vi "SMART__Yt13_SimpleGenericTest.vi"() -> ()   [LabVIEW 2017]
uses:
  Step`s VIs/YYLLIdea/yylltestresult/yylltestresult basis.ctl
  <vilib>/Utility/miscctls.llb/LVPointTypeDef.ctl
  <vilib>/Instr/_visa.llb/VISA Configure Serial Port (Instr).vi
panel:
  in  "Hex?(StringLimit-A)":bool caption="Hex?"
  in  "Hex?(接收解析后)":bool caption="Hex?"
  in  "Hex?(最终发送)":bool caption="Hex?"
  in  "真发送并获取接收的":bool
  in  "解析后到变量(自定义建议#开头)":string(combo)="不到变量"
  in  "明码LOG":bool
  in  "unit":string
  out "WaitTime":u32 format="%dms"
  in  "打开串口":bool
  in  "baud rate":string(combo)="9600"
  in  "应答≥长度检测":i32
  in  "应答检测":string
  in  "Hex?(假设接收)":bool caption="Hex?"
  out "结果预览":bool
  in  "LowLimit-C":dbl
  in  "UpperLimit-B":dbl
  in  "StringLimit-A":string
  in  "合格依据":T1 caption="Enum 3"
  in  "假设、收到的\n字符串":string
  out "解析后":string
  in  "Smart解析预处理btn":bool
  out "最终发送":string
  in  "发送字符串":string
  in  "Smart发送预处理btn":bool
  in  "Smart解析预处理":string[][](array[string])
  in  "Smart发送预处理":string[][](array[string])
  in  "VISA resource":refnum<visa-resource-name>
  in  "接收前延迟ms":u32
  in  "接收延迟前&发送前清缓存":bool=TRUE
  in  "Hex?(发送)":bool caption="Hex?"
  # "yyllSerial.SimpleTest"
  # "需提前运行好串口配置步骤！或这里临时打开"
  # "注意自收发参与统计"
  # "解析后：\nX值 ->"
  # "#yylltips:要判断MAC可以通过正则“\\w{12}”"
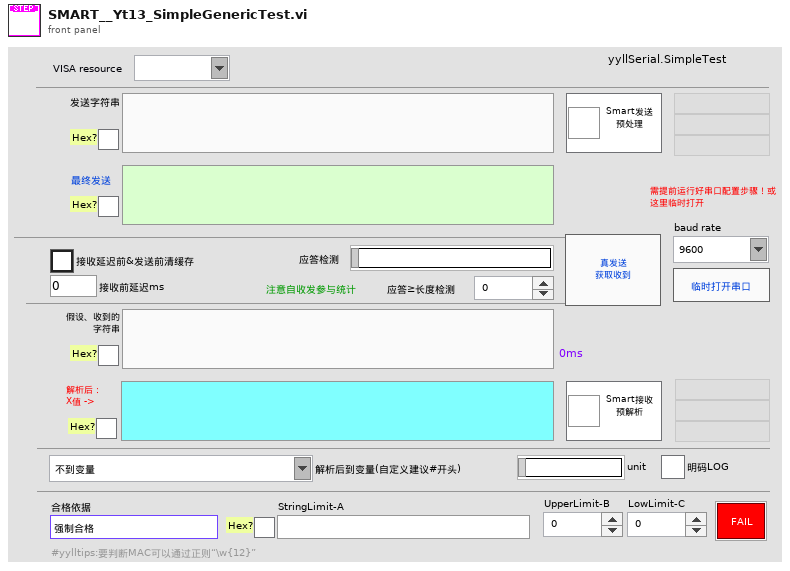
[diagram p1: front panel]
types:
  T1 = typedef "yylltestresult basis.ctl" = enum16{"强制合格", "强制不合格", "随机合格", "X=A", "X=\"真\"", "X=\"假\"", "X≠A", "X包含A", "X不包含A", "A包含X", "A包含非空X", "A不包含X", "X等于A正则匹配内容", "X包含A正则匹配内容", "X不包含A正则匹配内容", "X=B", "X≠B", "X＞B", "X≥B", "X＜B", "X≤B", "B≥X≥C", "B≥X＞C", "B＞X≥C", "B＞X＞C", "X≥B | C≥X", "X＞B | C≥X", "X≥B | C＞X", "X＞B | C＞X"}
  T2 = typedef "LVPointTypeDef.ctl" = cluster{"Horizontal":i16, "Vertical":i16}
  T3 = enum16{"open", "replace", "create", "open or create", "replace or create", "replace or create with confirmation"}
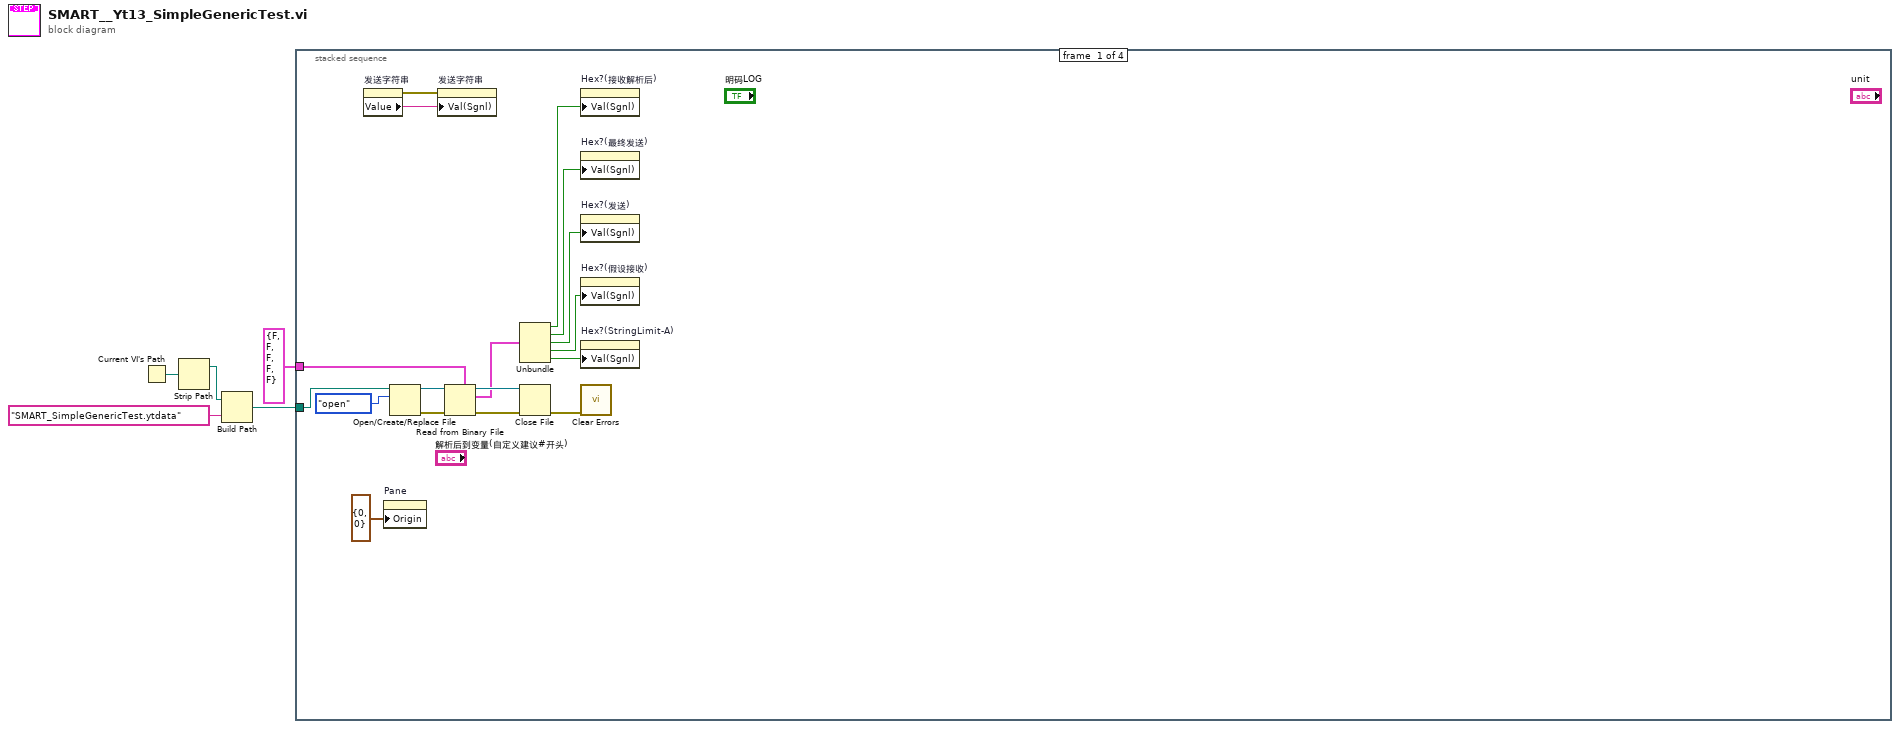
[diagram p0: block diagram]
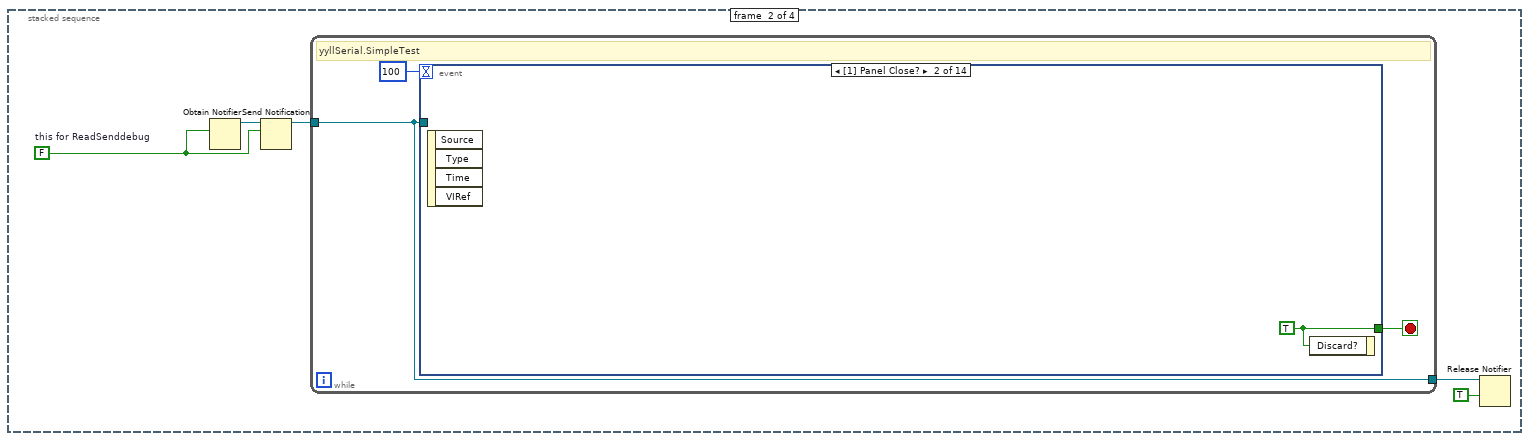
[diagram p2: hidden frame]
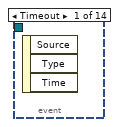
[diagram p3: hidden frame]
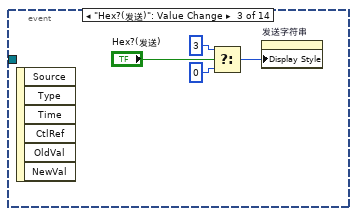
[diagram p4: hidden frame]
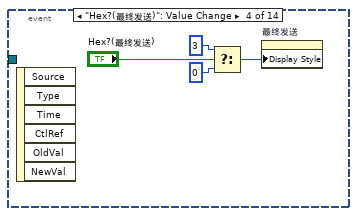
[diagram p5: hidden frame]
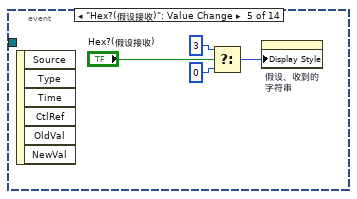
[diagram p6: hidden frame]
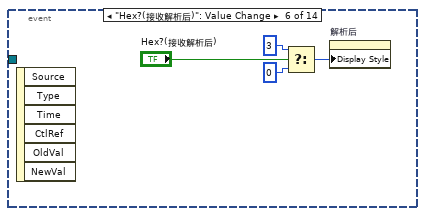
[diagram p7: hidden frame]
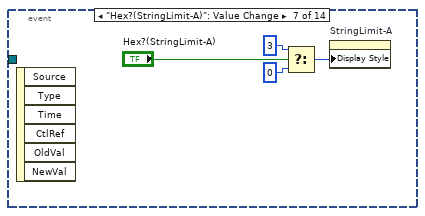
[diagram p8: hidden frame]
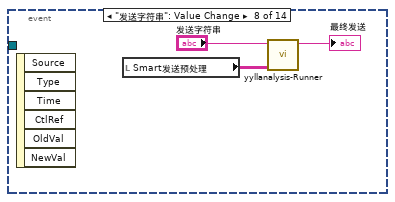
[diagram p9: hidden frame]
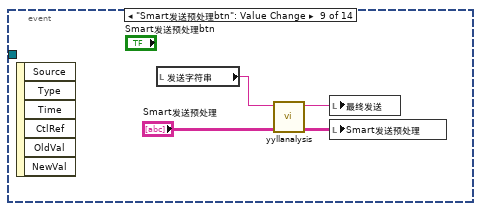
[diagram p10: hidden frame]
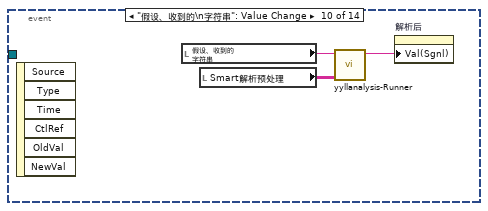
[diagram p11: hidden frame]
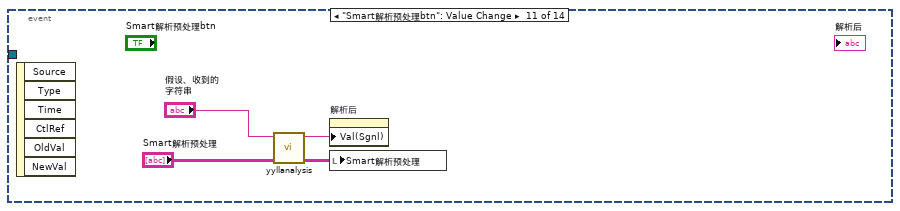
[diagram p12: hidden frame]
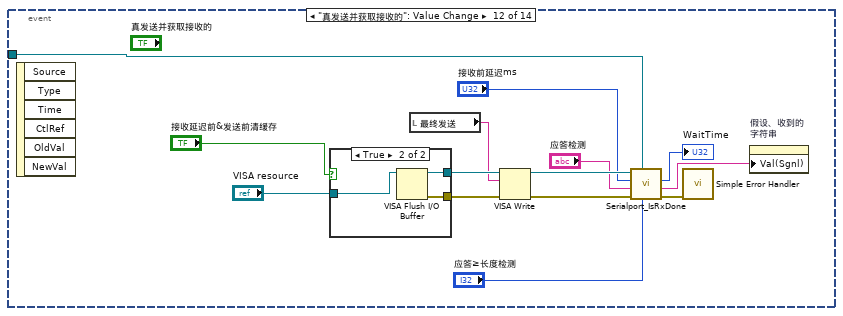
[diagram p13: hidden frame]
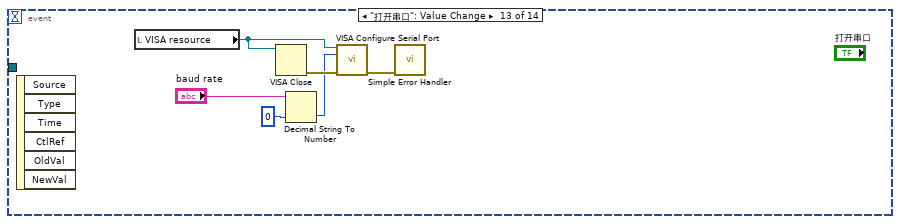
[diagram p15: hidden frame]
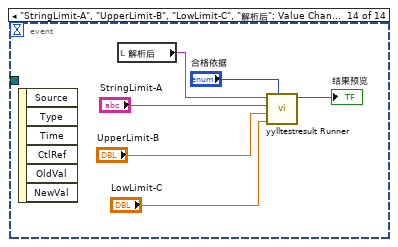
[diagram p16: hidden frame]
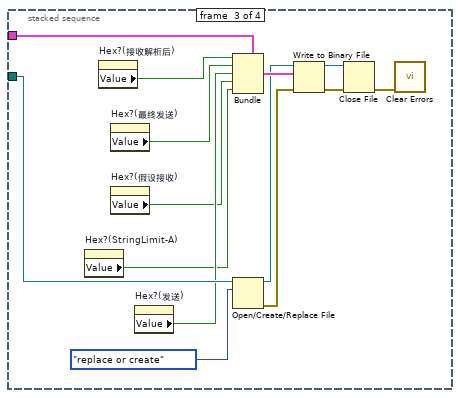
[diagram p17: hidden frame]
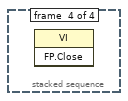
[diagram p18: hidden frame]
diagram:
  n1 = Current VI's Path() -> (path=w3:path)
  n2 = Strip Path(path=w3) -> (stripped path=w4:path)  [unwired: 1 out]
  n3 = Build Path(base path=w4, name or relative path="SMART_SimpleGenericTest.ytdata") -> (appended path=w2:path)
  n4 = stacked-sequence {
    tunnel: cluster{bool, bool, bool, bool, bool} {FALSE, FALSE, FALSE, FALSE, FALSE} -> [w9 _ w109 _]
    tunnel: w2 -> [w8 _ w108 _]
    frame #0 {
      n5 = property on="发送字符串" class="Str"() -> (error out=w22:errorcluster, "Value"=w21:string)  [unwired: 2 in, 1 out]
      n6 = property on="Pane" class="Pane"("Origin"=T2 {"Horizontal"=0, "Vertical"=0}) -> ()  [unwired: 2 in, 2 out]
      n7 = Open/Create/Replace File(file path (use dialog)=w8, operation (0:open)=T3."open") -> (refnum out=w12:refnum<file>, error out=w10:errorcluster)  [unwired: 4 in, 1 out]
      n8 = property on="发送字符串" class="Str"(error in=w22, "Val(Sgnl)"=w21) -> ()  [unwired: 1 in, 2 out]
      n9 = Read from Binary File(5:w9, 8:w10, 11:w12) -> (0:w13:errorcluster, 2:w14:cluster{bool, bool, bool, bool, bool}, 3:w20:refnum<file>)  [unwired: 3 in, 1 out]
      n10 = Unbundle(w14) -> (w19:bool, w18:bool, w17:bool, w16:bool, w15:bool)
      n11 = Close File(refnum=w20, error in=w13) -> (error out=w7:errorcluster)  [unwired: 1 out]
      n12 = property on="Hex?(接收解析后)" class="Bool (strict)"("Val(Sgnl)"=w19) -> ()  [unwired: 2 in, 2 out]
      n13 = property on="Hex?(最终发送)" class="Bool (strict)"("Val(Sgnl)"=w18) -> ()  [unwired: 2 in, 2 out]
      n14 = property on="Hex?(发送)" class="Bool (strict)"("Val(Sgnl)"=w17) -> ()  [unwired: 2 in, 2 out]
      n15 = property on="Hex?(假设接收)" class="Bool (strict)"("Val(Sgnl)"=w16) -> ()  [unwired: 2 in, 2 out]
      n16 = property on="Hex?(StringLimit-A)" class="Bool (strict)"("Val(Sgnl)"=w15) -> ()  [unwired: 2 in, 2 out]
      n17 = call <vilib>:"Clear Errors.vi"("error in (no error)"=w7) -> ()  [unwired: 5 in, 2 out]
    }
    frame #1 {
      w23 = FALSE  # this for ReadSenddebug
      n18 = Obtain Notifier(notification data type=w23) -> (notifier out=w25:refnum<notifier>)  [unwired: 3 in, 2 out]
      n19 = Send Notification(notification=w23, notifier=w25) -> (notifier out=w26:refnum<notifier>)  [unwired: 1 in, 1 out]
      n20 = while {
        tunnel: w26 -> [w28]
        tunnel: [w28] -> w27
        stop <- w29 stop-if-true
        # "yyllSerial.SimpleTest"
        n21 = event shown="[1] Panel Close?" {
          selector: _ -> [_ _ _ _ _ _ _ _ _ _ _ _ _ _]
          dyn-events: _ -> [_ _ _ _ _ _ _ _ _ _ _ _ _ _]
          timeout: 100 -> [_ _ _ _ _ _ _ _ _ _ _ _ _ _]
          tunnel: [_ w31 _ _ _ _ _ _ _ _ _ _ _ _] -> w29
          tunnel: w28 -> [_ _ _ _ _ _ _ _ _ _ _ w67 _ _]
          event Timeout {
            n22 = event-data() -> ()  [unwired: 1 in, 3 out]
          }
          event Panel Close? {
            w31 = TRUE
            n23 = event-data() -> ()  [unwired: 1 in, 4 out]
            n24 = event-data("Discard?"=w31) -> ()  [unwired: 1 in, 1 out]
          }
          event "Hex?(发送)": Value Change {
            n25 = event-data() -> ()  [unwired: 1 in, 6 out]
            n26 = Select(t=u32 3, s="Hex?(发送)", f=u32 0 ("Display Style")) -> (s? t:f=w32:u32)
            n27 = property on="发送字符串" class="Str"("Display Style"=w32) -> ()  [unwired: 2 in, 2 out]
          }
          event "Hex?(最终发送)": Value Change {
            n28 = event-data() -> ()  [unwired: 1 in, 6 out]
            n29 = Select(t=u32 3, s="Hex?(最终发送)", f=u32 0 ("Display Style")) -> (s? t:f=w38:u32)
            n30 = property on="最终发送" class="Str"("Display Style"=w38) -> ()  [unwired: 2 in, 2 out]
          }
          event "Hex?(假设接收)": Value Change {
            n31 = event-data() -> ()  [unwired: 1 in, 6 out]
            n32 = Select(t=u32 3, s="Hex?(假设接收)", f=u32 0 ("Display Style")) -> (s? t:f=w40:u32)
            n33 = property on="假设、收到的\n字符串" class="Str"("Display Style"=w40) -> ()  [unwired: 2 in, 2 out]
          }
          event "Hex?(接收解析后)": Value Change {
            n34 = event-data() -> ()  [unwired: 1 in, 6 out]
            n35 = Select(t=u32 3, s="Hex?(接收解析后)", f=u32 0 ("Display Style")) -> (s? t:f=w47:u32)
            n36 = property on="解析后" class="Str"("Display Style"=w47) -> ()  [unwired: 2 in, 2 out]
          }
          event "Hex?(StringLimit-A)": Value Change {
            n37 = event-data() -> ()  [unwired: 1 in, 6 out]
            n38 = Select(t=u32 3, s="Hex?(StringLimit-A)", f=u32 0 ("Display Style")) -> (s? t:f=w51:u32)
            n39 = property on="StringLimit-A" class="Str"("Display Style"=w51) -> ()  [unwired: 2 in, 2 out]
          }
          event "发送字符串": Value Change {
            n40 = event-data() -> ()  [unwired: 1 in, 6 out]
            n41 = local read "Smart发送预处理"() -> (w52:string[][])
            n42 = call "yyllanalysis-Runner.vi"("inputs"=w52, "String in"="发送字符串") -> ("String out"=→"最终发送":string)  [unwired: 8 in, 1 out]
          }
          event "Smart发送预处理btn": Value Change {
            n43 = event-data() -> ()  [unwired: 1 in, 6 out]
            n44 = local read "发送字符串"() -> (w56:string)
            n45 = call "yyllanalysis.vi"("Datain"="Smart发送预处理", "StringIN"=w56) -> ("Dataout"=w57:string[][], "StringOUT"=w55:string)  [unwired: 8 in]
            n46 = local write "最终发送"(w55) -> ()
            n47 = local write "Smart发送预处理"(w57) -> ()
          }
          event "假设、收到的\n字符串": Value Change {
            n48 = event-data() -> ()  [unwired: 1 in, 6 out]
            n49 = local read "假设、收到的\n字符串"() -> (w61:string)
            n50 = local read "Smart解析预处理"() -> (w60:string[][])
            n51 = call "yyllanalysis-Runner.vi"("inputs"=w60, "String in"=w61) -> ("String out"=w59:string)  [unwired: 8 in, 1 out]
            n52 = property on="解析后" class="Str"("Val(Sgnl)"=w59) -> ()  [unwired: 2 in, 2 out]
          }
          event "Smart解析预处理btn": Value Change {
            n53 = event-data() -> ()  [unwired: 1 in, 6 out]
            n54 = call "yyllanalysis.vi"("Datain"="Smart解析预处理", "StringIN"="假设、收到的\n字符串") -> ("Dataout"=w64:string[][], "StringOUT"=w62:string)  [unwired: 8 in]
            n55 = property on="解析后" class="Str"("Val(Sgnl)"=w62) -> ()  [unwired: 2 in, 2 out]
            n56 = local write "Smart解析预处理"(w64) -> ()
          }
          event "真发送并获取接收的": Value Change {
            n57 = event-data() -> ()  [unwired: 1 in, 6 out]
            n58 = case shown="True" "接收延迟前&发送前清缓存" {
              tunnel: "VISA resource" -> [w80 w83]
              tunnel: [w80 w82] -> w79
              tunnel: [_ w81] -> w78
              frame False {
              }
              frame True {
                n59 = VISA Flush I/O Buffer(VISA resource name=w83) -> (VISA resource name out=w82:refnum<visa-resource-name>, error out=w81:errorcluster)  [unwired: 2 in]
              }
            }
            n60 = local read "最终发送"() -> (w76:string)
            n61 = VISA Write(VISA resource name=w79, write buffer=w76, error in (no error)=w78) -> (VISA resource name out=w74:refnum<visa-resource-name>, error out=w70:errorcluster)  [unwired: 1 out]
            n62 = call "Serialport_IsRxDone.vi"("应答长度检测"="应答≥长度检测", "StopFlagRef"=w67, "error in (no error)"=w70, "应答检测"="应答检测", "接收前延迟ms"="接收前延迟ms", "VISA"=w74) -> ("error out"=w69:errorcluster, "Rx"=w68:string, "WaitTime"=→"WaitTime":u32)  [unwired: 2 in, 1 out]
            n63 = call <vilib>:"Simple Error Handler.vi"("error in (no error)"=w69) -> ()  [unwired: 4 in, 5 out]
            n64 = property on="假设、收到的\n字符串" class="Str"("Val(Sgnl)"=w68) -> ()  [unwired: 2 in, 2 out]
          }
          event "打开串口": Value Change {
            n65 = event-data() -> ()  [unwired: 1 in, 6 out]
            n66 = local read "VISA resource"() -> (w85:refnum<visa-resource-name>)
            n67 = VISA Close(VISA resource name=w85) -> (error out=w89:errorcluster)  [unwired: 1 in]
            n68 = Decimal String To Number(string="baud rate", default (0L)=u32 0 ("default (0 I32)")) -> (number=w86:u32)  [unwired: 1 in, 1 out]
            n69 = call-poly "VISA Configure Serial Port"("VISA resource name"=w85, "baud rate (9600)"=w86, "error in (no error)"=w89) -> ("error out"=w84:errorcluster)  [unwired: 11 in, 1 out]
            n70 = call <vilib>:"Simple Error Handler.vi"("error in (no error)"=w84) -> ()  [unwired: 4 in, 5 out]
          }
          event "StringLimit-A", "UpperLimit-B", "LowLimit-C", "解析后": Value Change {
            n71 = event-data() -> ()  [unwired: 1 in, 6 out]
            n72 = local read "解析后"() -> (w95:string)
            n73 = call "yylltestresult Runner.vi"("合格依据"="合格依据", "LowLimit-C"="LowLimit-C", "UpperLimit-B"="UpperLimit-B", "StringLimit-A"="StringLimit-A", "DataIn-X"=w95) -> ("isPass"=→"结果预览":bool)  [unwired: 4 in, 2 out]
          }
        }
      }
      n74 = Release Notifier(notifier=w27, force destroy? (F)=TRUE) -> ()  [unwired: 1 in, 3 out]
    }
    frame #2 {
      n75 = property on="Hex?(StringLimit-A)" class="Bool (strict)"() -> ("Value"=w103:bool)  [unwired: 2 in, 2 out]
      n76 = property on="Hex?(接收解析后)" class="Bool (strict)"() -> ("Value"=w107:bool)  [unwired: 2 in, 2 out]
      n77 = property on="Hex?(最终发送)" class="Bool (strict)"() -> ("Value"=w106:bool)  [unwired: 2 in, 2 out]
      n78 = property on="Hex?(假设接收)" class="Bool (strict)"() -> ("Value"=w104:bool)  [unwired: 2 in, 2 out]
      n79 = property on="Hex?(发送)" class="Bool (strict)"() -> ("Value"=w105:bool)  [unwired: 2 in, 2 out]
      n80 = Bundle(cluster=w109, w107, w106, w105, w104, w103) -> (w100:cluster{bool, bool, bool, bool, bool})
      n81 = Open/Create/Replace File(file path (use dialog)=w108, operation (0:open)=T3."replace or create") -> (refnum out=w99:refnum<file>, error out=w98:errorcluster)  [unwired: 4 in, 1 out]
      n82 = Write to Binary File(file (use dialog)=w99, data=w100, error in=w98) -> (refnum out=w102:refnum<file>, error out=w101:errorcluster)  [unwired: 3 in, 1 out]
      n83 = Close File(refnum=w102, error in=w101) -> (error out=w96:errorcluster)  [unwired: 1 out]
      n84 = call <vilib>:"Clear Errors.vi"("error in (no error)"=w96) -> ()  [unwired: 5 in, 2 out]
    }
    frame #3 {
      n85 = invoke class="VI" method="FP.Close"() -> ()  [unwired: 3 in, 3 out]
    }
  }
